vi "GetElapsedTime.vi"(1 "Start Time":timestamp) -> (0 "Elapsed Time [s]":sgl)   [LabVIEW 2017]
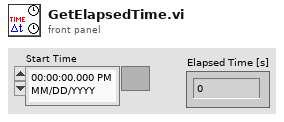
[diagram p1: front panel]
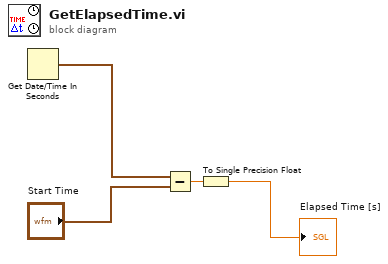
[diagram p0: block diagram]
diagram:
  n1 = Get Date/Time In Seconds() -> (seconds since 1Jan1904=w3:timestamp)
  n2 = Subtract(x=w3, y="Start Time") -> (x-y=w4:dbl)
  n3 = To Single Precision Float(number=w4) -> (single precision float=→"Elapsed Time [s]":sgl)
